vi "Create Input Signal.vi"(8 "error in (no error)":errorcluster, 10 "Signal Parameters":T2 {"Byte Order" items=["Little Endian", "Big Endian"]; "Data Type" items=["Signed", "Unsigned", "IEEE Float"]}, 11 "Section Ptr":T1 format="%.0x") -> (0 "error out":errorcluster, 3 "Section Ptr out":T1 format="%.0x")   [LabVIEW 2015, in "Diagnostics Addon System Explorer.lvlib"]
uses:
  System Explorer/Diagnostics Addon System Explorer.lvlib
  Signal Parameters.ctl
  <vilib>/NI Veristand/Custom Device API/Custom Device Item Ref.ctl
  <vilib>/NI Veristand/Custom Device API/Custom Device Channel.ctl
  <vilib>/NI Veristand/Custom Device API/Custom Device Channel Type.ctl
  FG Action.ctl
  <vilib>/NI Veristand/Custom Device API/NI VeriStand - Get Item Property.vi
  <vilib>/NI Veristand/Custom Device API/Get Item Property (String).vi
  <vilib>/NI Veristand/Custom Device API/Get Item Property (Double).vi
  <vilib>/NI Veristand/Custom Device API/Get Item Property (U32).vi
  <vilib>/NI Veristand/Custom Device API/NI VeriStand - Set Item Property.vi
  <vilib>/NI Veristand/Custom Device API/Set Item Property (String).vi
  <vilib>/NI Veristand/Custom Device API/Set Item Property (Double).vi
  <vilib>/NI Veristand/Custom Device API/Set Item Property (U32).vi
  GUID Lookup.vi
  <vilib>/NI Veristand/Custom Device API/Custom Device API.lvlib
  Diagnostics Addon Shared.lvlib
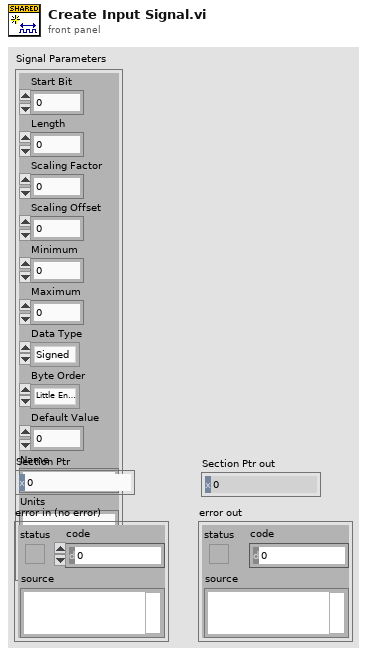
[diagram p1: front panel]
types:
  T1 = typedef "Custom Device API.lvlib/Custom Device Item Ref.ctl" = u64
  T2 = typedef "Diagnostics Addon Shared.lvlib/Signal Parameters.ctl" = cluster{"Start Bit":u8, "Length":u8, "Scaling Factor":dbl, "Scaling Offset":dbl, "Minimum":dbl, "Maximum":dbl, "Data Type":u32, "Byte Order":u32, "Default Value":dbl, "Name":string, "Units":string, "Description":string}
  T3 = typedef "Diagnostics Addon System Explorer.lvlib/FG Action.ctl" = enum16{"Get", "Set"}
  T4 = typedef "Custom Device API.lvlib/Custom Device Channel.ctl" = cluster{"Type":T5, "Units":string, "Default Value":dbl, "Faultable":bool, "Scalable":bool}
  T5 = typedef "Custom Device API.lvlib/Custom Device Channel Type.ctl" = enum16{"Input", "Output"}
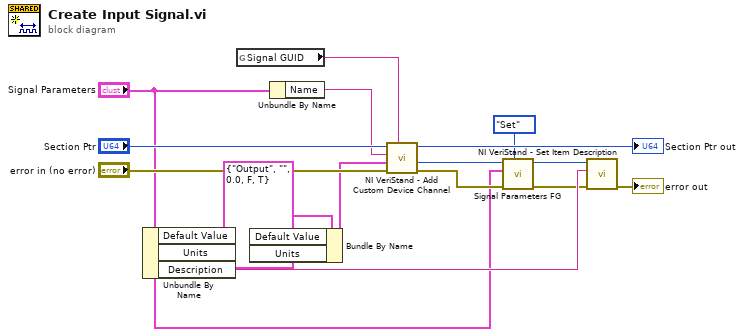
[diagram p0: block diagram]
diagram:
  n1 = Unbundle By Name("Signal Parameters") -> ("Default Value"=w11:dbl, "Units"=w10:string, "Description"=w7:string)
  n2 = global read "GUID Lookup.vi" "Signal GUID"() -> (w13:string)
  n3 = Bundle By Name(cluster=T4 {"Type"=enum."Output", "Units"="", "Default Value"=0.0, "Faultable"=FALSE, "Scalable"=TRUE} ("Channel"), "Default Value"=w11, "Units"=w10) -> (w8:T4)
  n4 = Unbundle By Name("Signal Parameters") -> ("Name"=w16:string)
  n5 = call <vilib>:"NI VeriStand - Add Custom Device Channel.vi"("GUID (Default Channel)"=w13, "error in (no error)"="error in (no error)", "Channel"=w8, "Channel Name"=w16, "Parent Ref in"="Section Ptr") -> ("error out"=w5:errorcluster, "Channel Ref"=w3:T1, "Parent Ref out"=→"Section Ptr out":T1)  [unwired: 3 in, 1 out]
  n6 = call "Signal Parameters FG.vi"("Action"=FG_Action."Set", "error in (no error)"=w5, "Signal Parameters"="Signal Parameters", "Device Item Ref in"=w3) -> ("error out"=w4:errorcluster, "Device Item Ref out"=w2:T1)  [unwired: 5 in, 1 out]
  n7 = call <vilib>:"NI VeriStand - Set Item Description.vi"("error in (no error)"=w4, "Description"=w7, "Item Ref in"=w2) -> ("error out"=→"error out":errorcluster)  [unwired: 6 in, 2 out]
